vi "Move_3_axis_linear_Peregrine.vi"(0 "Handle in":refnum<visa-resource-name>, 1 "Address x":u8, 2 "Address y":u8, 3 "Address z":u8, 5 "Target x":i32, 7 "Target y":i32, 9 "Target z":i32, 11 "error":errorcluster, 12 "Speed":i16, 14 "Acceleration":u16) -> (4 "Handle out":refnum<visa-resource-name>, 15 "error out":errorcluster)   [LabVIEW 2019]
panel:
  out "dz":i32
  out "Position z":i32
  out "dx":i32
  out "dy":i32
  out "Position y":i32
  out "Position x":i32
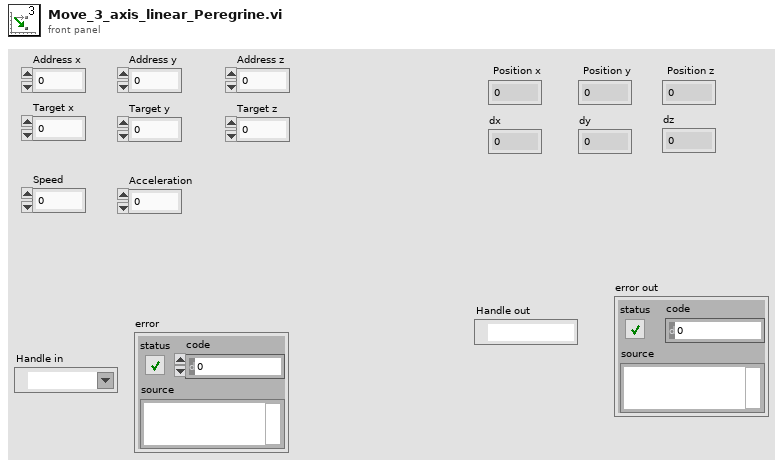
[diagram p1: front panel]
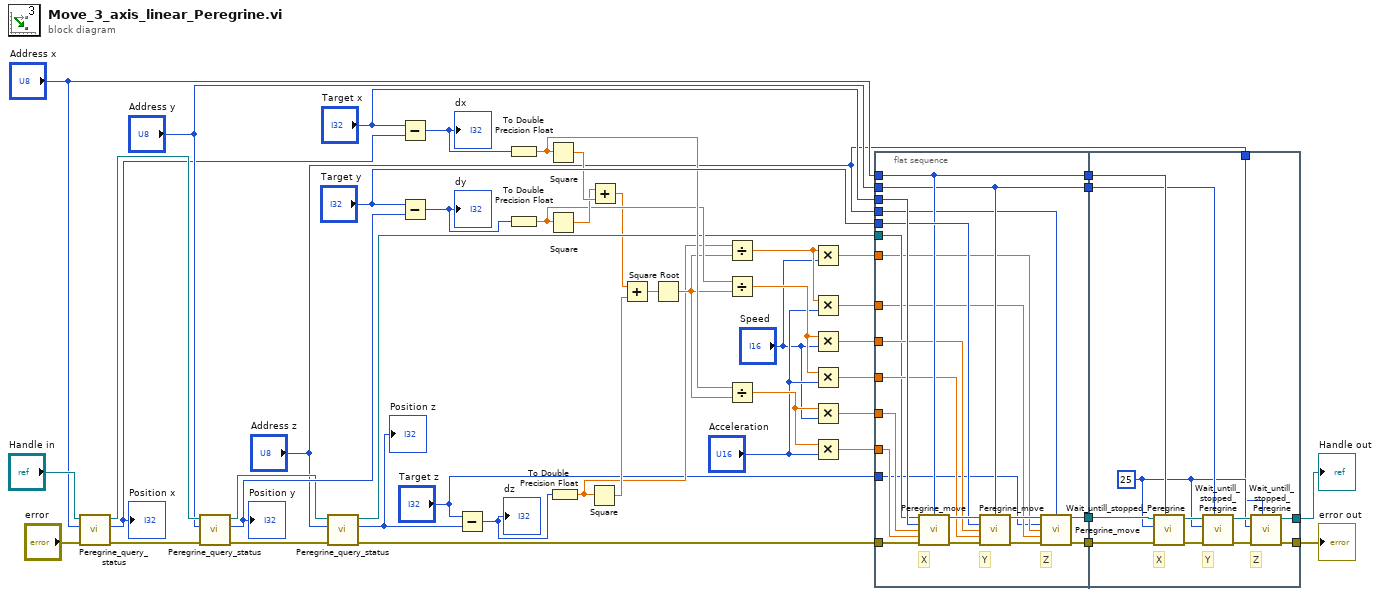
[diagram p0: block diagram]
diagram:
  n1 = call "Peregrine_query_status.vi"("error"="error", "Address"="Address x", "Handle in"="Handle in") -> ("error out"=w39:errorcluster, "Position"=w33:i32, "Handle out"=w40:refnum<visa-resource-name>)  [unwired: 4 in, 2 out]
  "Position x" <- w33
  n2 = call "Peregrine_query_status.vi"("error"=w39, "Address"="Address y", "Handle in"=w40) -> ("error out"=w17:errorcluster, "Position"=w32:i32, "Handle out"=w18:refnum<visa-resource-name>)  [unwired: 4 in, 2 out]
  "Position y" <- w32
  n3 = call "Peregrine_query_status.vi"("error"=w17, "Address"="Address z", "Handle in"=w18) -> ("error out"=w15:errorcluster, "Position"=w14:i32, "Handle out"=w16:refnum<visa-resource-name>)  [unwired: 4 in, 2 out]
  "Position z" <- w14
  n4 = Subtract(x="Target x", y=w33) -> (x-y=w30:i32)
  "dx" <- w30
  n5 = Subtract(x="Target y", y=w32) -> (x-y=w29:i32)
  "dy" <- w29
  n6 = Subtract(x="Target z", y=w14) -> (x-y=w13:i32)
  "dz" <- w13
  n7 = To Double Precision Float(number=w30) -> (double precision float=w26:dbl)
  n8 = To Double Precision Float(number=w29) -> (double precision float=w25:dbl)
  n9 = Square(x=w26) -> (x^2=w28:dbl)
  n10 = Square(x=w25) -> (x^2=w27:dbl)
  n11 = To Double Precision Float(number=w13) -> (double precision float=w8:dbl)
  n12 = Square(x=w8) -> (x^2=w11:dbl)
  n13 = Add(x=w27, y=w28) -> (x+y=w12:dbl)
  n14 = Add(x=w12, y=w11) -> (x+y=w10:dbl)
  n15 = Square Root(x=w10) -> (sqrt(x)=w9:dbl)
  n16 = Divide(x=w8, y=w9) -> (x/y=w7:dbl)
  n17 = Divide(x=w25, y=w9) -> (x/y=w23:dbl)
  n18 = Divide(x=w26, y=w9) -> (x/y=w21:dbl)
  n19 = Multiply(x=w7, y="Speed") -> (x*y=w3:dbl)
  n20 = Multiply(x=w7, y="Acceleration") -> (x*y=w4:dbl)
  n21 = Multiply(x=w23, y="Speed") -> (x*y=w22:dbl)
  n22 = Multiply(x=w23, y="Acceleration") -> (x*y=w24:dbl)
  n23 = Multiply(x=w21, y="Speed") -> (x*y=w20:dbl)
  n24 = Multiply(x=w21, y="Acceleration") -> (x*y=w19:dbl)
  n25 = flat-sequence {
    tunnel: "Address x" -> [w62]
    tunnel: "Target x" -> [w66]
    tunnel: [w54] -> w46
    tunnel: [w53] -> w45
    tunnel: "Target y" -> [w63]
    tunnel: [w62] -> w42
    tunnel: "Address y" -> [w61]
    tunnel: [w61] -> w41
    tunnel: w24 -> [w60]
    tunnel: w22 -> [w59]
    tunnel: w20 -> [w58]
    tunnel: w19 -> [w57]
    tunnel: w16 -> [w52]
    tunnel: w15 -> [w51]
    tunnel: w4 -> [w50]
    tunnel: w3 -> [w49]
    tunnel: "Target z" -> [w48]
    tunnel: "Address z" -> [w47]
    tunnel: w46 -> [w78]
    tunnel: w45 -> [w77]
    tunnel: [w70] -> w44
    tunnel: [w69] -> w43
    tunnel: w42 -> [w74]
    tunnel: w41 -> [w73]
    tunnel: "Address z" -> [w67]
    frame #0 {
      # "Z"
      # "Y"
      # "X"
      n26 = call "Peregrine_move.vi"("Handle in"=w52, "Address"=w62, "Target"=w66, "Speed"=w58, "Acceleration"=w57, "error"=w51) -> ("Handle out"=w65:refnum<visa-resource-name>, "error out"=w64:errorcluster)  [unwired: 8 in]
      n27 = call "Peregrine_move.vi"("Handle in"=w65, "Address"=w61, "Target"=w63, "Speed"=w59, "Acceleration"=w60, "error"=w64) -> ("Handle out"=w56:refnum<visa-resource-name>, "error out"=w55:errorcluster)  [unwired: 8 in]
      n28 = call "Peregrine_move.vi"("Handle in"=w56, "Address"=w47, "Target"=w48, "Speed"=w49, "Acceleration"=w50, "error"=w55) -> ("Handle out"=w54:refnum<visa-resource-name>, "error out"=w53:errorcluster)  [unwired: 8 in]
    }
    frame #1 {
      w68 = u32 25 ("milliseconds to wait")
      # "Z"
      # "Y"
      # "X"
      n29 = call "Wait_untill_stopped_Peregrine.vi"("Address"=w74, "error"=w77, "milliseconds to wait"=w68, "Handle in"=w78) -> ("error out"=w75:errorcluster, "Handle out"=w76:refnum<visa-resource-name>)  [unwired: 2 in, 4 out]
      n30 = call "Wait_untill_stopped_Peregrine.vi"("Address"=w73, "error"=w75, "milliseconds to wait"=w68, "Handle in"=w76) -> ("error out"=w71:errorcluster, "Handle out"=w72:refnum<visa-resource-name>)  [unwired: 2 in, 4 out]
      n31 = call "Wait_untill_stopped_Peregrine.vi"("Address"=w67, "error"=w71, "milliseconds to wait"=w68, "Handle in"=w72) -> ("error out"=w69:errorcluster, "Handle out"=w70:refnum<visa-resource-name>)  [unwired: 2 in, 4 out]
    }
  }
  "Handle out" <- w44
  "error out" <- w43
